vi "errcode.vi"(8 "error in (no error)":errorcluster, 11 "db":dbl) -> (0 "error out":errorcluster, 2 "function return":i32, 3 "db out":dbl)   [LabVIEW 2020, in "sqlite3.lvlib"]
uses:
  sqlite3.lvlib
  errstr.vi
  bin/sqlite3_64.dll
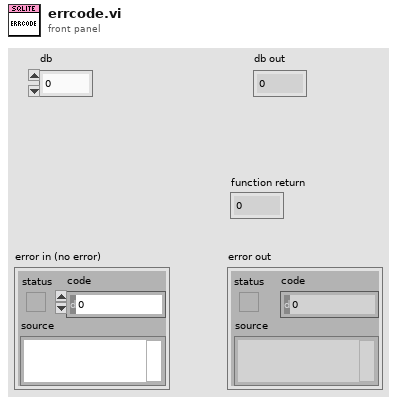
[diagram p1: front panel]
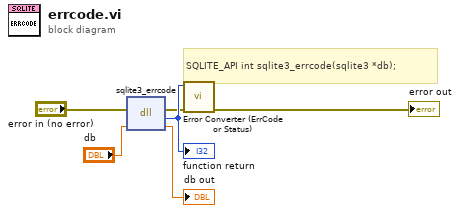
[diagram p0: block diagram]
diagram:
  # "SQLITE_API int sqlite3_errcode(sqlite3 *db);"
  n1 = dll-call lib="D:/Project/Labview-Projects/database-configuration/externals/sqlite3/Source/bin/sqlite3_*.*" fn="sqlite3_errcode"(error in="error in (no error)", "db"="db") -> (error out=w2:errorcluster, w6:i32, "db"=→"db out":dbl)  [unwired: 2 in, 1 out]
  "function return" <- w6
  n2 = call "Error Converter (ErrCode or Status).vi"("error in (no error)"=w2, "error code"=w6) -> ("error out"=→"error out":errorcluster)  [unwired: 9 in]
